vi "LoadedScript_Execution.vi"(8 "error in (no error)":errorcluster, 11 "Script of MS Process":string) -> (0 "error out":errorcluster)   [LabVIEW 2018]
uses:
  MSScript/MSScript.lvclass
  MSEncoder/MSEncoder.lvclass
panel:
  in  "Dialogue":i32(listbox)=-1
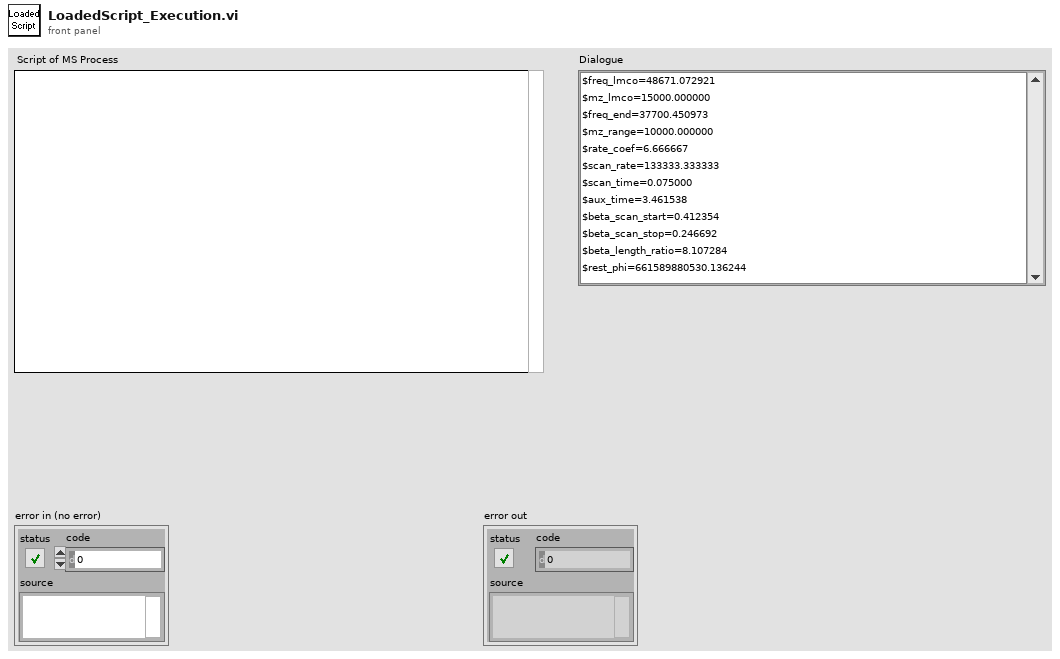
[diagram p1: front panel]
types:
  T1 = cluster{"Freq":ext, "Amp":ext, "Decyc":u32, "1/Decyc":u32, "MaxAmp":ext}
  T2 = cluster{"param":cluster{"label":string, "data":string}[], "code":string}
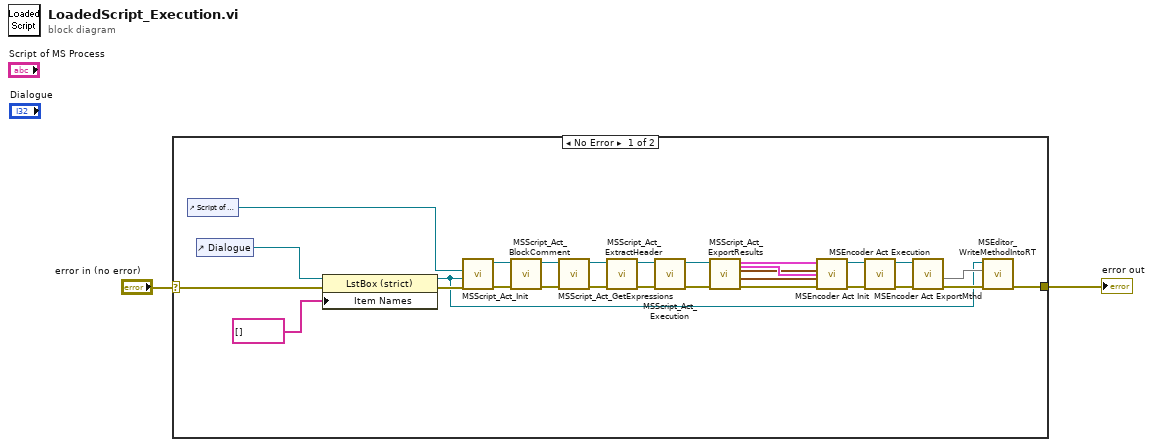
[diagram p0: block diagram]
diagram:
  n1 = case shown="No Error" "error in (no error)" {
    selector: "error in (no error)" -> [w3 w31]
    tunnel: [w11 w31] -> w2
    frame No Error {
      n2 = control-ref of="Script of MS Process"() -> (w22:refnum<vi>)
      n3 = control-ref of="Dialogue"() -> (w21:refnum<vi>)
      n4 = property class="LstBox (strict)"(reference=w21, error in=w3, "Item Names"=string[] []) -> (reference out=w12:refnum<vi>, error out=w19:errorcluster)
      n5 = call "MSScript_Act_Init.vi"("error in (no error)"=w19, "Listbox Ref"=w12, "Script ctl ref"=w22) -> ("error out"=w29:errorcluster, "MSScript out"=w30:refnum<class "MSScript.lvclass">)  [unwired: 7 in]
      n6 = call "MSScript_Act_BlockComment.vi"("error in (no error)"=w29, "MSScript in"=w30) -> ("error out"=w27:errorcluster, "MSScript out"=w28:refnum<class "MSScript.lvclass">)  [unwired: 8 in]
      n7 = call-dynamic "MSScript_Act_GetExpressions.vi"("error in (no error)"=w27, "MSScript in"=w28) -> ("error out"=w23:errorcluster, "MSScript out"=w24:refnum<class "MSScript.lvclass">)  [unwired: 8 in]
      n8 = call-dynamic "MSScript_Act_ExtractHeader.vi"("error in (no error)"=w23, "MSScript in"=w24) -> ("error out"=w25:errorcluster, "MSScript out"=w26:refnum<class "MSScript.lvclass">)  [unwired: 8 in]
      n9 = call-dynamic "MSScript_Act_Execution.vi"("error in (no error)"=w25, "MSScript in"=w26) -> ("error out"=w5:errorcluster, "MSScript out"=w6:refnum<class "MSScript.lvclass">)  [unwired: 8 in]
      n10 = call-dynamic "MSScript_Act_ExportResults.vi"("error in (no error)"=w5, "MSScript in"=w6) -> ("error out"=w4:errorcluster, "Ion trap"=w7:cluster{"R0":ext, "Z0":ext}, "PriRF"=w8:T1, "MS Process fmts"=w10:cluster{"Name":string, "Data":variant}[], "Script out"=w9:T2)  [unwired: 5 in]
      n11 = call "MSEncoder Act Init.vi"(5:w9, "error in (no error)"=w4, 7:w7, "scriptPythonCode"=w8, "eventProcess"=w10) -> ("error out"=w18:errorcluster, "MSEncoder out"=w15:refnum<class "MSEncoder.lvclass">)  [unwired: 3 in]
      n12 = call-dynamic "MSEncoder Act Execution.vi"("error in (no error)"=w18, "MSEncoder in"=w15) -> ("error out"=w17:errorcluster, "MSEncoder out"=w16:refnum<class "MSEncoder.lvclass">)  [unwired: 8 in]
      n13 = call-dynamic "MSEncoder Act ExportMthd.vi"("error in (no error)"=w17, "MSEncoder in"=w16) -> ("error out"=w13:errorcluster, 1:w14)  [unwired: 7 in, 1 out]
      n14 = call "MSEditor_WriteMethodIntoRT.vi"("error in"=w13, "Mthd in"=w14, "listbox ref in"=w12) -> ("error out"=w11:errorcluster)  [unwired: 7 in, 1 out]
    }
    frame Error {
    }
  }
  "error out" <- w2
